vi "RCV CAN data.vi"() -> ()   [LabVIEW 2016]
doc: "This is a practical example of CAN_READ.\nOn the left hand side of the BD is a disabled code section. One can enable this to log CAN data.\nThe potput of this disabled code segment is the error cluster.\nThan the selected channel will be initiatlized.\nOnce the initialisation is OK a timed while loop will be executed until CAN_READ will signal an error.\nInside of the while loop is the CAN_READ function.\nBuilding up an array of CAN mesages and timestamps is done while this loop executes.\nOnly the last message witch is naturaly empty, because the receive queue is empty, will be ignored.\nThe result is an array of received CAN messages."
uses:
  CAN Communication.llb/TPCANHandle.ctl
  CAN Communication.llb/TPCANBaudrate.ctl
  CAN Communication.llb/CAN MSG Cluster.ctl
  CAN Communication.llb/TPCANTimestampFD.ctl
  CAN Communication.llb/TPCANParameter.ctl
  <vilib>/Platform/TimedLoop/XDataNode/timing_clust.ctl
  <vilib>/Platform/TimedLoop/XDataNode/nitl_modes.ctl
  <vilib>/Platform/TimedLoop/XDataNode/wakeup.ctl
  CAN Communication.llb/PCAN Get CHANNEL CONDITION.vi
  <vilib>/Platform/TimedLoop/XDataNode/XDataNode.xnode
  <vilib>/Platform/TimedLoop/XDataNode/XDNodeRunTimeDep.lvlib
panel:
  out "TPCANMessageType out Strings":string
  out "CAN Timestamp":T1[](array[typedef]) format="%016x"
  out "CAN Data":T2[](array[typedef]) {"MSG type" format="%x"; "ID" format="%.0x"}
  in  "Release all channels first":bool=TRUE
  in  "TPCANBaudrate":T3
  in  "TPCANHandle":T4=enum."PCAN_USBBUS2  0x52"
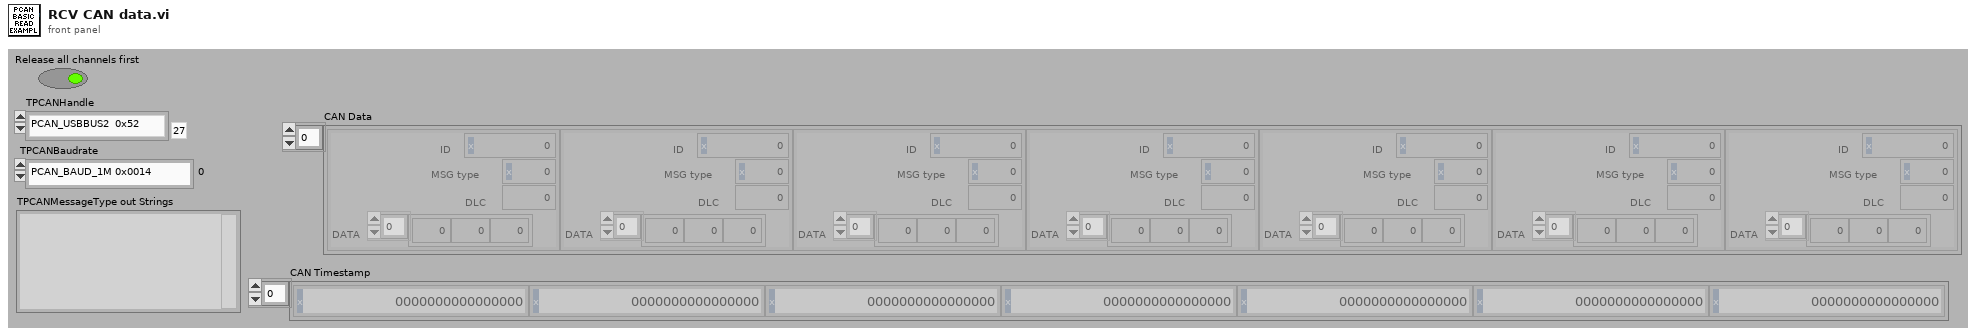
[diagram p1: front panel]
types:
  T1 = typedef "TPCANTimestampFD.ctl" = u64
  T2 = typedef "CAN MSG Cluster.ctl" = cluster{"ID":u32, "MSG type":u8, "DLC":u8, "DATA":u8[]}
  T3 = typedef "TPCANBaudrate.ctl" = enum16{"PCAN_BAUD_1M 0x0014", "PCAN_BAUD_800K 0x0016", "PCAN_BAUD_500K 0x001C", "PCAN_BAUD_250K 0x011C", "PCAN_BAUD_125K 0x031C", "PCAN_BAUD_100K 0x432F", "PCAN_BAUD_95K 0xC34E", "PCAN_BAUD_83K 0x852B", "PCAN_BAUD_50K 0x472F", "PCAN_BAUD_47K 0x1414", "PCAN_BAUD_33K 0x8B2F", "PCAN_BAUD_20K 0x532F", "PCAN_BAUD_10K 0x672F", "PCAN_BAUD_5K 0x7F7F", "User Baudrate"}
  T4 = typedef "TPCANHandle.ctl" = enum16{"PCAN_NONEBUS  0x000", "PCAN_ISABUS1  0x21", "PCAN_ISABUS2  0x22", "PCAN_ISABUS3  0x23", "PCAN_ISABUS4  0x24", "PCAN_ISABUS5  0x25", "PCAN_ISABUS6  0x26", "PCAN_ISABUS7  0x27", "PCAN_ISABUS8  0x28", "PCAN_DNGBUS1  0x31", "PCAN_PCIBUS1  0x41", "PCAN_PCIBUS1  0x42", "PCAN_PCIBUS1  0x43", "PCAN_PCIBUS1  0x44", "PCAN_PCIBUS1  0x45", "PCAN_PCIBUS1  0x46", "PCAN_PCIBUS1  0x47", "PCAN_PCIBUS1  0x48", "PCAN_PCIBUS1  0x409", "PCAN_PCIBUS1  0x40A", "PCAN_PCIBUS1  0x40B", "PCAN_PCIBUS1  0x40C", "PCAN_PCIBUS1  0x40D", "PCAN_PCIBUS1  0x40E", "PCAN_PCIBUS1  0x40F", "PCAN_PCIBUS1  0x410", "PCAN_USBBUS1  0x51", "PCAN_USBBUS2  0x52", "PCAN_USBBUS3  0x53", "PCAN_USBBUS4  0x54", "PCAN_USBBUS5  0x55", "PCAN_USBBUS6  0x56", "PCAN_USBBUS7  0x57", "PCAN_USBBUS8  0x58", "PCAN_USBBUS9  0x509", "PCAN_USBBUS10  0x50A", "PCAN_USBBUS11  0x50B", "PCAN_USBBUS12  0x50C", "PCAN_USBBUS13  0x50D", "PCAN_USBBUS14  0x50E", "PCAN_USBBUS15  0x50F", "PCAN_USBBUS16  0x510", "PCAN_PCCBUS1  0x61", "PCAN_PCCBUS2  0x62", "PCAN_LANBUS1  0x801", "PCAN_LANBUS2  0x802", "PCAN_LANBUS3  0x803", "PCAN_LANBUS4  0x804", "PCAN_LANBUS5  0x805", "PCAN_LANBUS6  0x806", "PCAN_LANBUS7  0x807", "PCAN_LANBUS8  0x808", "PCAN_LANBUS9  0x809", "PCAN_LANBUS10  0x80A", "PCAN_LANBUS11  0x80B", "PCAN_LANBUS12  0x80C", "PCAN_LANBUS13  0x80D", "PCAN_LANBUS14  0x80E", "PCAN_LANBUS15  0x80F", "PCAN_LANBUS16  0x810"}
  T5 = typedef "TPCANParameter.ctl" = enum8{"Not Available", "PCAN device number", "PCAN 5-volt power", "PCAN receive event", "PCAN message filter", "PCAN API version", "PCAN channel version", "PCAN busoff autoreset", "PCAN listen-only", "PCAN log location", "PCAN log status", "PCAN log configure", "PCAN log text", "PCAN channel condition", "PCAN hardware name", "PCAN_RECEIVE_STATUS", "PCAN_CONTROLLER_NUMBER", "PCAN_TRACE_LOCATION ", "PCAN_TRACE_STATUS", "PCAN_TRACE_SIZE", "PCAN_TRACE_CONFIGURE", "PCAN_CHANNEL_IDENTIFYING", "PCAN_CHANNEL_FEATURES", "PCAN_SPEED_ADAPTING", "PCAN_BITRATE_INFO", "PCAN_BITRATE_INFO_FD", "PCAN_BUSSPEED_NOMINAL", "PCAN_BUSSPEED_DATA", "PCAN_IP_ADDRESS", "PCAN_LAN_SERVICE_STATUS", "PCAN_ALLOW_STATUS_FRAMES", "PCAN_ALLOW_RTR_FRAMES", "PCAN_ALLOW_ERROR_FRAMES", "PCAN_INTERFRAME_DELAY", "PCAN_ACCEPTANCE_FILTER_11BIT", "PCAN_ACCEPTANCE_FILTER_29BIT", "PCAN_IO_DIGITAL_CONFIGURATION", "PCAN_IO_DIGITAL_VALUE", "PCAN_IO_DIGITAL_SET", "PCAN_IO_DIGITAL_CLEAR", "PCAN_IO_ANALOG_VALUE"}
  T6 = typedef "Channel Availability.ctl" = enum16{"PCAN_CHANNEL_UNAVAILABLE", "PCAN_CHANNEL_AVAILABLE", "PCAN_CHANNEL_OCCUPIED"}
  T7 = typedef "XDNodeRunTimeDep.lvlib/timing_clust.ctl" = cluster{"Expected End [f-1]":u64, "Actual End [f-1]":u64, "Finished Late? [f-1]":bool, "Expected End [i-1]":u64, "Actual End [i-1]":u64, "Finished Late? [i-1]":bool, "Expected Start [i]":u64, "Actual Start [i]":u64, "Expected Start [f]":u64, "Actual Start [f]":u64, "Source Name":string, "Structure Name":string, "Period":i64, "Deadline":i64, "Offset":i64, "Start":i64, "Priority":i32, "Timeout":i32, "Mode":T8, "Wakeup Reason":T9, "Error":errorcluster, "Source Type":string, "Secondary Source Type":string, "Global End Time":u64, "Global Start Time":u64, "Frame Duration":u64, "Iteration Duration":u64, "Assigned CPU":i32, "I/O Scan Engine Mode":u32}
  T8 = typedef "XDNodeRunTimeDep.lvlib/nitl_modes.ctl" = enum32{"No Change", "Process missed periods, maintain original phase", "Discard missed periods, maintain original phase", "Process missed periods, ignore original phase", "Discard missed periods, ignore original phase"}
  T9 = typedef "XDNodeRunTimeDep.lvlib/wakeup.ctl" = enum32{"Normal", "Aborted", "Asynchronous wakeup", "Timing source error", "Timed loop error", "Timeout"}
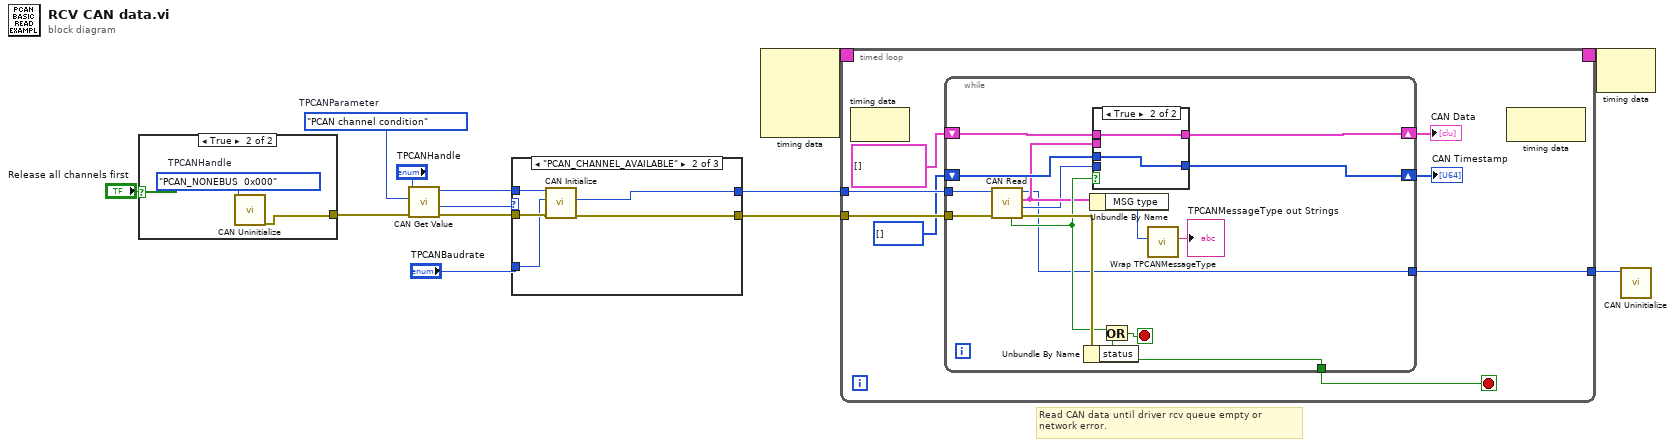
[diagram p0: block diagram]
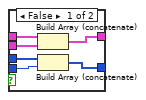
[diagram p2: hidden frame]
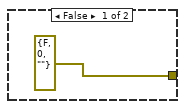
[diagram p3: hidden frame]
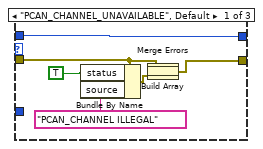
[diagram p4: hidden frame]
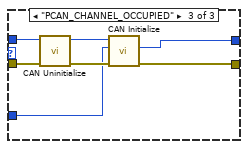
[diagram p5: hidden frame]
diagram:
  w13 = TPCANParameter."PCAN channel condition"  # TPCANParameter
  # "Read CAN data until driver rcv queue empty or\nnetwork error."
  n1 = case shown="True" "Release all channels first" {
    tunnel: [errorcluster {"status"=FALSE, "code"=0, "source"=""} ("error out") w16] -> w7
    frame False {
    }
    frame True {
      w15 = TPCANHandle."PCAN_NONEBUS  0x000"  # TPCANHandle
      n2 = call "CAN Uninitialize.vi"("TPCANHandle"=w15) -> ("error out"=w16:errorcluster)  [unwired: 8 in, 2 out]
    }
  }
  n3 = call-poly "CAN Get Value.vi"("error in (no error)"=w7, "TPCANParameter"=w13, "TPCANHandle"="TPCANHandle") -> ("error out"=w10:errorcluster, "Channel condition"=w9:T6, "TPCANHandle out"=w11:T4)  [unwired: 6 in]
  n4 = case shown="\"PCAN_CHANNEL_AVAILABLE\"" w9 {
    tunnel: [w22 w28 w32] -> w4
    tunnel: w11 -> [w23 w27 w34]
    tunnel: w10 -> [w21 w26 w35]
    tunnel: "TPCANBaudrate" -> [_ w24 w29]
    tunnel: [w23 w25 w30] -> w5
    frame "PCAN_CHANNEL_UNAVAILABLE", Default {
      n5 = Bundle By Name(cluster=w21, "status"=TRUE, "source"="PCAN_CHANNEL ILLEGAL") -> (w18:errorcluster)
      n6 = Build Array(w21, w18) -> (w17:errorcluster[])
      n7 = Merge Errors(w17) -> (w22:errorcluster)
    }
    frame "PCAN_CHANNEL_AVAILABLE" {
      n8 = call "CAN Initialize.vi"("error in (no error)"=w26, "TPCANBaudrate"=w24, "TPCANHandle"=w27) -> ("error out"=w28:errorcluster, "TPCANHandle_out"=w25:T4)  [unwired: 6 in, 1 out]
    }
    frame "PCAN_CHANNEL_OCCUPIED" {
      n9 = call "CAN Uninitialize.vi"("error in (no error)"=w35, "TPCANHandle"=w34) -> ("error out"=w33:errorcluster, "TPCANHandle out"=w31:T4)  [unwired: 7 in, 1 out]
      n10 = call "CAN Initialize.vi"("error in (no error)"=w33, "TPCANBaudrate"=w29, "TPCANHandle"=w31) -> ("error out"=w32:errorcluster, "TPCANHandle_out"=w30:T4)  [unwired: 6 in, 1 out]
    }
  }
  n11 = node-c288() -> (w3:T7)  [unwired: 4 in]
  n12 = timed-loop {
    timing: w3 -> [_]
    timing-out: [_] -> w2
    tunnel: w5 -> [w43]
    tunnel: w4 -> [w42]
    tunnel: [w36] -> w1
    stop <- w41 stop-if-true
    n13 = node-c288() -> ()  [unwired: 1 in, 1 out]
    n14 = while {
      tunnel: w43 -> [w58]
      tunnel: w42 -> [w57]
      tunnel: [w54] -> w41
      shift-right: [w51] -> w40
      shift-left: T2[] [] -> [w52]
      shift-right: [w49] -> w37
      shift-left: u64[] [] -> [w50]
      tunnel: [w44] -> w36
      stop <- w55 stop-if-true
      n15 = call "CAN Read.vi"("error in (no error)"=w57, "TPCANHandle"=w58) -> ("error out"=w56:errorcluster, "TPCANTimestamp out"=w45:T1, "CAN_Message out"=w48:T2, "TPCANHandle out"=w44:T4, "rcv queue empty"=w53:bool)  [unwired: 5 in]
      n16 = Unbundle By Name(w56) -> ("status"=w54:bool)
      n17 = Unbundle By Name(w48) -> ("MSG type"=w47:u8)
      n18 = case shown="True" w53 {
        tunnel: w52 -> [w64 w66]
        tunnel: [w63 w66] -> w51
        tunnel: w48 -> [w62 _]
        tunnel: w50 -> [w61 w65]
        tunnel: w45 -> [w60 _]
        tunnel: [w59 w65] -> w49
        frame False {
          n19 = Build Array (concatenate)(w64, w62) -> (w63:T2[])
          n20 = Build Array (concatenate)(w61, w60) -> (w59:T1[])
        }
        frame True {
        }
      }
      n21 = Or(x=w53, y=w54) -> (x .or. y?=w55:bool)
      n22 = call "Wrap TPCANMessageType.vi"("TPCANMessageType Numeric"=w47) -> ("TPCANMessageType out Strings"=→"TPCANMessageType out Strings":string)  [unwired: 9 in, 1 out]
    }
    "CAN Data" <- w40
    "CAN Timestamp" <- w37
    n23 = node-c288() -> ()  [unwired: 1 in, 1 out]
  }
  n24 = node-c288(w2) -> ()  [unwired: 1 out]
  n25 = call "CAN Uninitialize.vi"("TPCANHandle"=w1) -> ()  [unwired: 8 in, 3 out]
